vi "publishEventILCCommunication.vi"(8 "error in (no error)":errorcluster, 11 "Model in":refnum<class "Model.lvclass">) -> (0 "error out":errorcluster, 3 "Model out":refnum<class "Model.lvclass">)   [LabVIEW 2016, in "Model.lvclass"]
uses:
  Model.lvclass
  Model.lvclass/Model.ctl
  ILCCommunications/ILCCommunications.lvclass/ILCCommunications.ctl
  Publisher/Publisher.lvclass/Publisher.ctl
  Communicator/M1M3SAL/M1M3SAL.lvclass/M1M3SAL.ctl
  Publisher/getM1M3SAL.vi
  Publisher/setM1M3SAL.vi
  Communicator/M1M3SAL/logILCCommunication.vi
  Publisher/getLastPublishedTimeoutActuatorIds.vi
  Publisher/setLastPublishedTimeoutActuatorIds.vi
  Communicator/M1M3SAL/writeHeader.vi
  Communicator/M1M3SAL/writeDBL.vi
  Communicator/M1M3SAL/writeI32.vi
  Communicator/M1M3SAL/writeBoolean.vi
  Communicator/M1M3SAL/writeU8.vi
  ILCCommunications/ILCCommunications.lvclass
  Publisher/Publisher.lvclass
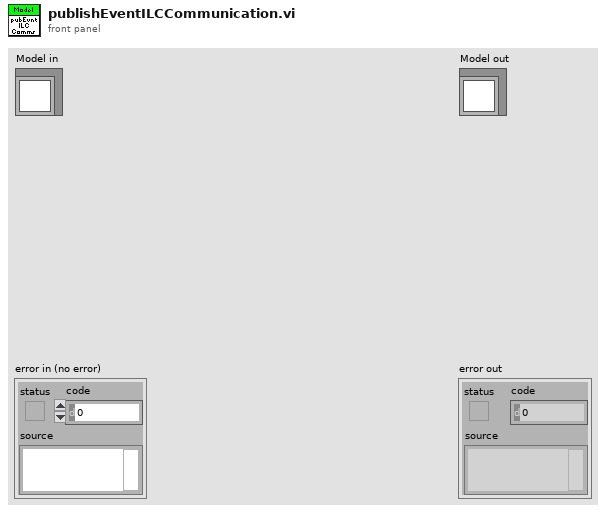
[diagram p1: front panel]
types:
  T1 = typedef "M1M3SupportTopics.lvlib/Timestamp.ctl" = dbl
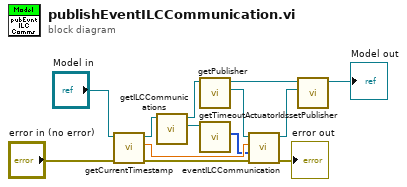
[diagram p0: block diagram]
diagram:
  n1 = call "getCurrentTimestamp.vi"("error in (no error)"="error in (no error)", "Model in"="Model in") -> ("error out"=w2:errorcluster, "Timestamp"=w7:T1, "Model out"=w10:refnum<class "Model.lvclass">)  [unwired: 7 in]
  n2 = call "getILCCommunications.vi"("Model in"=w10) -> ("ILCCommunications"=w9:refnum<class "ILCCommunications.lvclass">, "Model out"=w5:refnum<class "Model.lvclass">)  [unwired: 9 in]
  n3 = call "getPublisher.vi"("Model in"=w5) -> ("Publisher"=w8:refnum<class "Publisher.lvclass">, "Model out"=w13:refnum<class "Model.lvclass">)  [unwired: 9 in]
  n4 = call "getTimeoutActuatorIds.vi"("ILCCommunications in"=w9) -> ("TimeoutActuatorIds"=w6:i32[])  [unwired: 9 in, 1 out]
  n5 = call "eventILCCommunication.vi"("error in (no error)"=w2, "TimeoutActuatorIds"=w6, "Timestamp"=w7, "Publisher in"=w8) -> ("error out"=→"error out":errorcluster, "Publisher out"=w4:refnum<class "Publisher.lvclass">)  [unwired: 6 in]
  n6 = call "setPublisher.vi"("Publisher"=w4, "Model in"=w13) -> ("Model out"=→"Model out":refnum<class "Model.lvclass">)  [unwired: 9 in]
